vi "CThread Core.vi"   [LabVIEW 2012, in "CThread.lvlib"]
uses:
  CThread.lvlib
  XNodes/initializernode/CThread Initializer.xnode
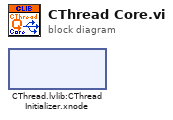
[diagram p0: block diagram]
diagram:
  n1 = xnode "CThread.lvlib:CThread Initializer.xnode"() -> ()
